vi "Set Class Instance.vi"(11 "TypeOsciloscope":string) -> (3 "Name":refnum<class "OsciloscopeClass.lvclass">)   [LabVIEW 2020]
uses:
  Class/OsciloscopeClass/OsciloscopeClass.lvclass
panel:
  out "Classes":string[](array[string])
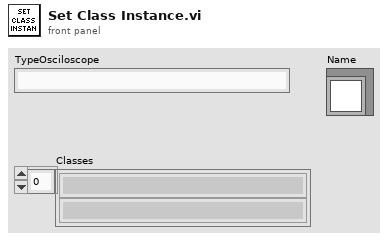
[diagram p1: front panel]
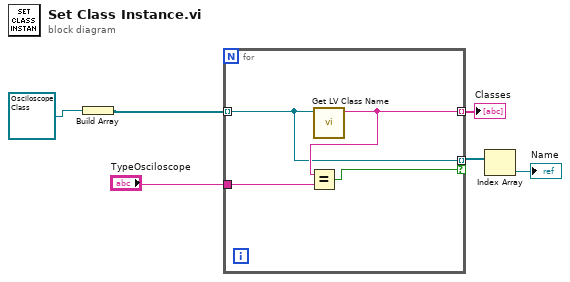
[diagram p0: block diagram]
diagram:
  n1 = Build Array(refnum<class "OsciloscopeClass.lvclass"> refnum ("OsciloscopeClass.lvclass")) -> (w3:refnum<class "OsciloscopeClass.lvclass">[])
  n2 = for {
    tunnel: w3 -> [w8] mode=indexing
    tunnel: [w9] -> w6 mode=indexing
    tunnel: "TypeOsciloscope" -> [w10]
    tunnel: [w8] -> w4 mode=indexing if=w7
    n3 = call <vilib>:"Get LV Class Name.vi"("object"=w8) -> ("class name"=w9:string)  [unwired: 9 in, 1 out]
    n4 = Equal?(x=w9, y=w10) -> (x = y?=w7:bool)
  }
  "Classes" <- w6
  n5 = Index Array(array=w4) -> (element=→"Name":refnum<class "OsciloscopeClass.lvclass">)  [unwired: 1 in]
